vi "Read_Transducer_Array.vi"(8 "error in (no error)":errorcluster, 10 "Pressure Range Array":dbl[](array[numeric])) -> (0 "error out":errorcluster, 1 "Timing (ms)":u32, 2 "Pressure Output":dbl[](array[numeric]))   [LabVIEW 2019]
panel:
  in  "Pressure init Array":dbl[](array[numeric])=[10.0, 10.0, 10.0, 10.0, 10.0, 10.0, 10.0, 0.00395164]
  out "appended array":dbl[](array[numeric])
  # "Read all NI 9203 Channels"
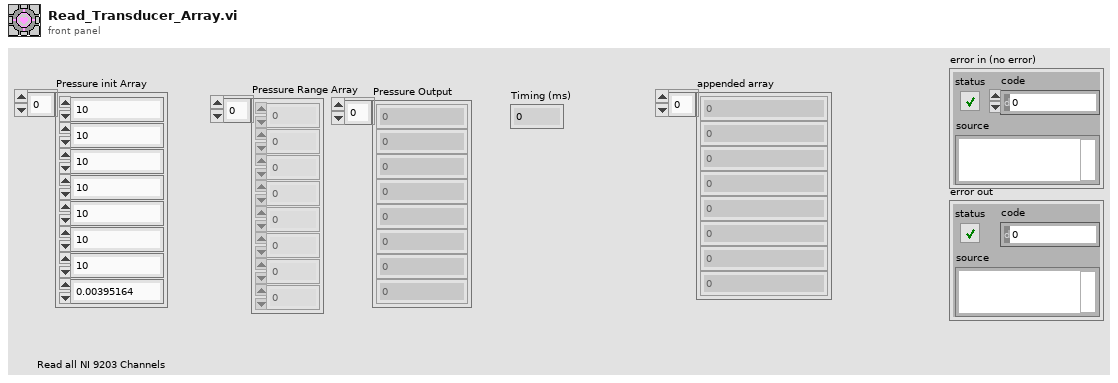
[diagram p1: front panel]
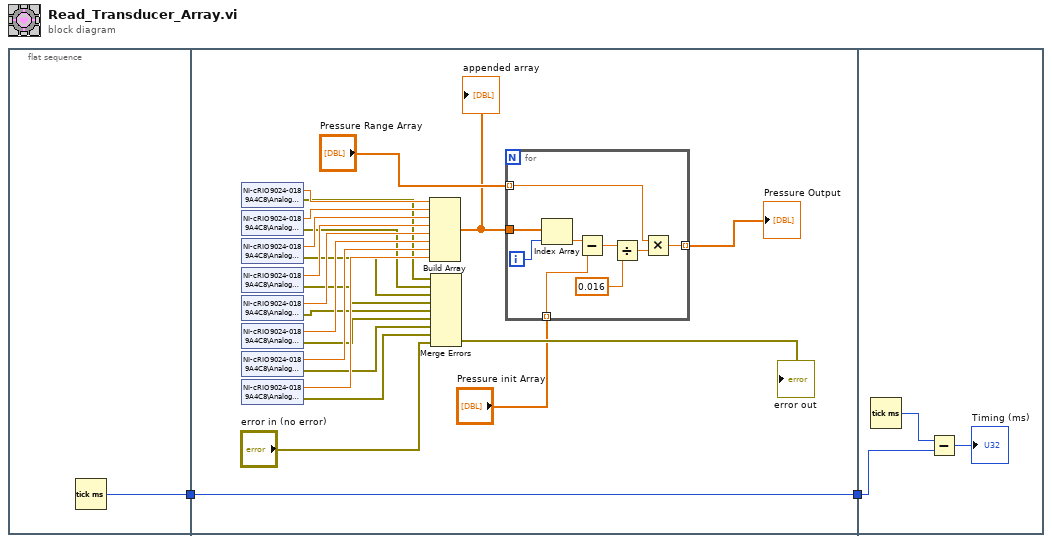
[diagram p0: block diagram]
diagram:
  n1 = flat-sequence {
    tunnel: [w3] -> w1
    tunnel: [w5] -> w2
    tunnel: w1 -> [w5]
    tunnel: w2 -> [w37]
    frame #0 {
      n2 = Tick Count (ms)() -> (millisecond timer value=w3:u32)
    }
    frame #1 {
      n3 = shared-variable "NI-cRIO9024-0189A4C8\\Analog Current In\\AI0"() -> (w24:dbl, error out=w17:errorcluster)  [unwired: 1 in]
      n4 = shared-variable "NI-cRIO9024-0189A4C8\\Analog Current In\\AI1"() -> (w25:dbl, error out=w16:errorcluster)  [unwired: 1 in]
      n5 = shared-variable "NI-cRIO9024-0189A4C8\\Analog Current In\\AI2"() -> (w23:dbl, error out=w15:errorcluster)  [unwired: 1 in]
      n6 = shared-variable "NI-cRIO9024-0189A4C8\\Analog Current In\\AI3"() -> (w22:dbl, error out=w14:errorcluster)  [unwired: 1 in]
      n7 = shared-variable "NI-cRIO9024-0189A4C8\\Analog Current In\\AI4"() -> (w21:dbl, error out=w13:errorcluster)  [unwired: 1 in]
      n8 = shared-variable "NI-cRIO9024-0189A4C8\\Analog Current In\\AI5"() -> (w20:dbl, error out=w12:errorcluster)  [unwired: 1 in]
      n9 = shared-variable "NI-cRIO9024-0189A4C8\\Analog Current In\\AI6"() -> (w19:dbl, error out=w11:errorcluster)  [unwired: 1 in]
      n10 = shared-variable "NI-cRIO9024-0189A4C8\\Analog Current In\\AI7"() -> (w18:dbl, error out=w10:errorcluster)  [unwired: 1 in]
      n11 = Build Array(w24, w25, w23, w22, w21, w20, w19, w18) -> (w9:dbl[])
      "appended array" <- w9
      n12 = Merge Errors(w17, w16, w15, w14, w13, w12, w11, w10, "error in (no error)") -> (→"error out":errorcluster)
      n13 = for {
        tunnel: "Pressure Range Array" -> [w29] mode=indexing
        tunnel: w9 -> [w35]
        tunnel: [w28] -> w8 mode=indexing
        tunnel: "Pressure init Array" -> [w27] mode=indexing
        i -> [w34]
        n14 = Index Array(array=w35, index=w34) -> (element=w33:dbl)
        n15 = Subtract(x=w33, y=w27) -> (x-y=w32:dbl)
        n16 = Divide(x=w32, y=0.016) -> (x/y=w30:dbl)
        n17 = Multiply(x=w29, y=w30) -> (x*y=w28:dbl)
      }
      "Pressure Output" <- w8
    }
    frame #2 {
      n18 = Tick Count (ms)() -> (millisecond timer value=w38:u32)
      n19 = Subtract(x=w38, y=w37) -> (x-y=→"Timing (ms)":u32)
    }
  }
